vi "GOES Message to Bit String.vi"(11 "GOES Message IN":string="CA99999321-@A@E_a@Q@B@@@@@_??BT@@@X_@f?v@O^M@@@@@@+?KV?jp@^@@V@Y@T+?@P?Rv@_P@U@X@S+~?r?S|@^^@U@X@S+~yv?JZ@bb@U@X@S+~?r?QR@aH@U@X@S") -> (0 "Boolean Byte Array OUT":bool[][](array[boolean]), 2 "Station ID":string, 3 "Decoded Bit String":string)   [LabVIEW 2016]
panel:
  out "resulting string":string
  out "Array":string[](array[string])
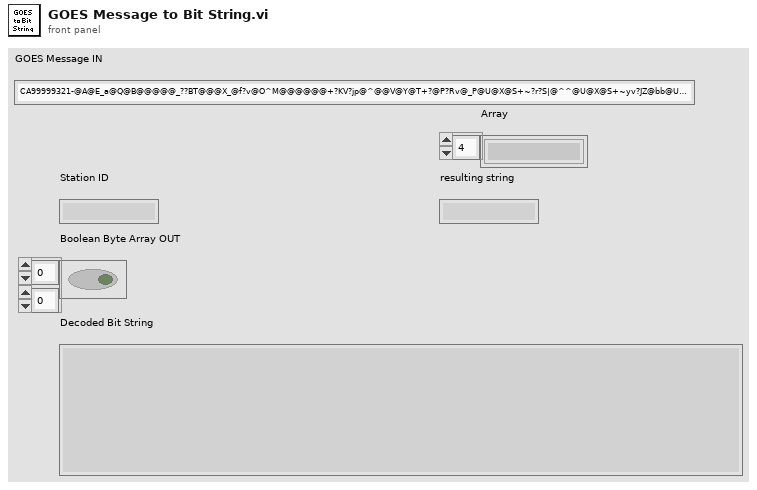
[diagram p1: front panel]
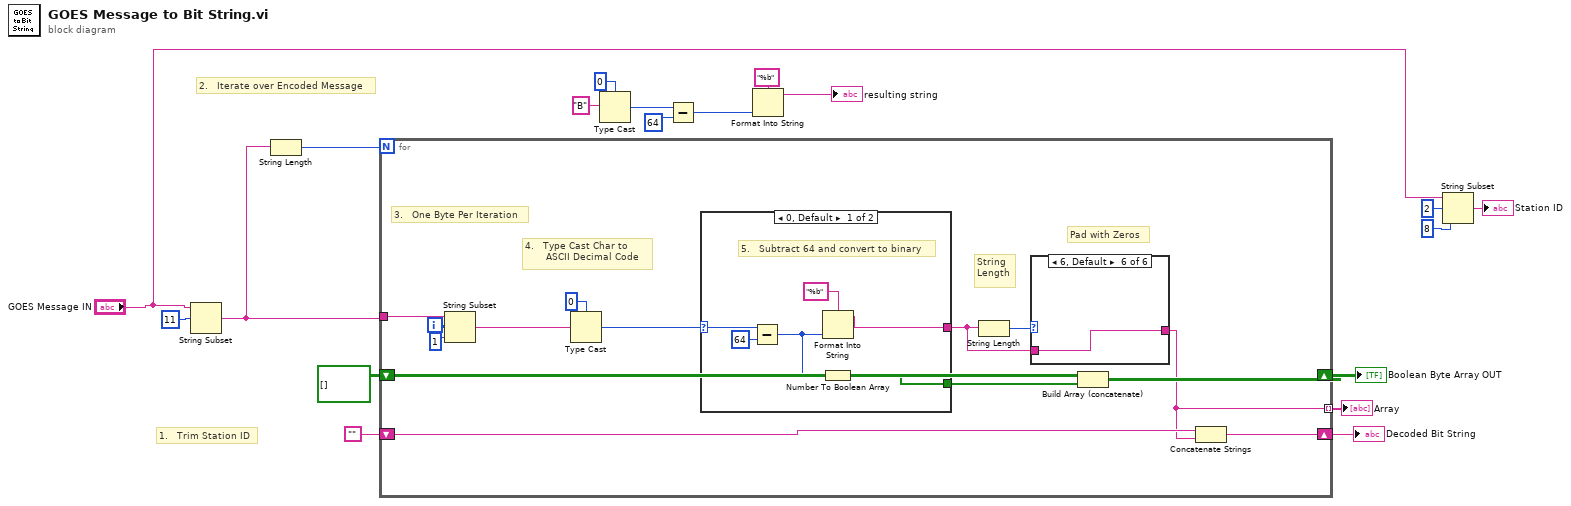
[diagram p0: block diagram]
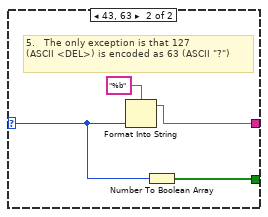
[diagram p2: hidden frame]
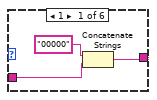
[diagram p3: hidden frame]
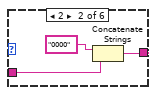
[diagram p4: hidden frame]
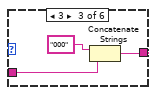
[diagram p5: hidden frame]
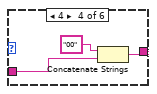
[diagram p6: hidden frame]
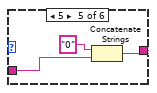
[diagram p7: hidden frame]
diagram:
  # "2.   Iterate over Encoded Message"
  # "1.   Trim Station ID"
  n1 = String Subset(string="GOES Message IN", offset (0)=11) -> (substring=w11:string)  [unwired: 1 in]
  n2 = String Length(string=w11) -> (length=w10:i32)
  n3 = for {
    N: w10 -> [_]
    tunnel: w11 -> [w33]
    shift-right: [w25] -> w13
    shift-left: bool[][] [] -> [w23]
    shift-right: [w21] -> w16
    shift-left: "" -> [w22]
    tunnel: [w20] -> w8 mode=indexing
    i -> [w32]
    # "Pad with Zeros"
    # "String\nLength"
    # "4.   Type Cast Char to \n       ASCII Decimal Code"
    # "3.   One Byte Per Iteration"
    n4 = String Subset(string=w33, offset (0)=w32, length (rest)=1 ("length (rest)")) -> (substring=w30:string)
    n5 = Type Cast(type=u8 0, x=w30) -> (*(type *) &x=w27:u8)
    n6 = case shown="0, Default" w27 {
      selector: w27 -> [w38 w41]
      tunnel: [w36 w40] -> w26
      tunnel: [w34 w43] -> w24
      frame 0, Default {
        # "5.   Subtract 64 and convert to binary"
        n7 = Subtract(x=w38, y=u8 64) -> (x-y=w35:u8)
        n8 = Format Into String(format string="%b", w35) -> (resulting string=w36:string)  [unwired: 2 in, 1 out]
        n9 = Number To Boolean Array(number=w35) -> (Boolean array=w34:bool[])
      }
      frame 43, 63 {
        # "5.   The only exception is that 127\n(ASCII <DEL>) is encoded as 63 (ASCII \"?\")"
        n10 = Format Into String(format string="%b", w41) -> (resulting string=w40:string)  [unwired: 2 in, 1 out]
        n11 = Number To Boolean Array(number=w41) -> (Boolean array=w43:bool[])
      }
    }
    n12 = String Length(string=w26) -> (length=w28:i32)
    n13 = case shown="6, Default" w28 {
      tunnel: w26 -> [w45 w48 w51 w54 w58 w59]
      tunnel: [w44 w47 w50 w53 w57 w59] -> w20
      frame 1 {
        n14 = Concatenate Strings("00000" ("string"), w45) -> (w44:string)
      }
      frame 2 {
        n15 = Concatenate Strings("0000" ("string"), w48) -> (w47:string)
      }
      frame 3 {
        n16 = Concatenate Strings("000" ("string"), w51) -> (w50:string)
      }
      frame 4 {
        n17 = Concatenate Strings("00" ("string"), w54) -> (w53:string)
      }
      frame 5 {
        n18 = Concatenate Strings("0" ("string"), w58) -> (w57:string)
      }
      frame 6, Default {
      }
    }
    n19 = Build Array (concatenate)(w23, w24) -> (w25:bool[][])
    n20 = Concatenate Strings(w22, w20) -> (w21:string)
  }
  "Decoded Bit String" <- w16
  "Boolean Byte Array OUT" <- w13
  "Array" <- w8
  n21 = Type Cast(type=u8 0, x="B" ("format string")) -> (*(type *) &x=w3:u8)
  n22 = Subtract(x=w3, y=u8 64) -> (x-y=w2:u8)
  n23 = Format Into String(format string="%b", w2) -> (resulting string=→"resulting string":string)  [unwired: 2 in, 1 out]
  n24 = String Subset(string="GOES Message IN", offset (0)=2, length (rest)=8 ("offset (0)")) -> (substring=→"Station ID":string)
